vi "MeasuringDevice.UnInit.vi"(8 "error in (no error)":errorcluster, 11 "MeasuringDevice":refnum<class "MeasuringDevice.lvclass">) -> (0 "error out":errorcluster, 3 "MeasuringDevice out":refnum<class "MeasuringDevice.lvclass">)   [LabVIEW 2017, in "MeasuringDevice.lvclass"]
doc: "---------------------------------------------------------------\nJKI State Machine Objects™\nhttp://jki.net/state-machine-objects/\nCopyright (C) 2005-2015, JKI <info@jki.net>\nALL RIGHTS RESERVEDJKI State Machine Objects (SMO) 1.0.0.5\nJKI - JKI\nCopyright (c) 2016, JKI"
uses:
  MeasuringDevice.lvclass
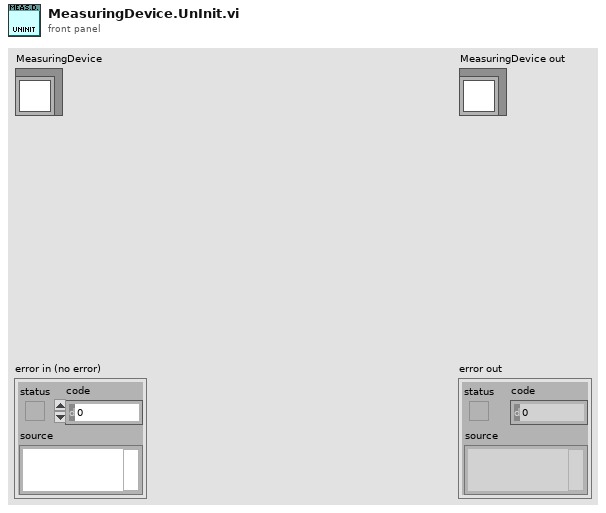
[diagram p1: front panel]
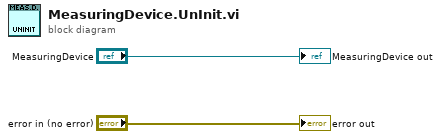
[diagram p0: block diagram]
diagram:
  "error out" <- "error in (no error)"
  "MeasuringDevice out" <- "MeasuringDevice"
